vi "GaussianPeakFinder.vi"(3 "Mode":T4, 5 "Traverse line In":T1 {"Row Duration (mins)" format="%#.1f"; "Row No" min=0; "Trace Gas Concentration (%)" min=0.0 format="%#.2f"; "Emission Rate (l/min)" format="%#.2f"; "Tunnel Speed" format="%#.2f"; "Start X" format="%#.2f"; "Start Y" format="%#.2f"; "Start Z" format="%#.2f"; "End X" format="%#.2f"; "End Y" format="%#.2f"; "End Z" format="%#.2f"; "Averaging time (min)" min=0.0 format="%#.2f"}) -> (0 "Error Message":string, 1 "Status":T5, 2 "Traverse line Out":T1 {"Row Duration (mins)" format="%#.1f"; "Row No" min=0; "Trace Gas Concentration (%)" min=0.0 format="%#.2f"; "Emission Rate (l/min)" format="%#.2f"; "Tunnel Speed" format="%#.2f"; "Start X" format="%#.2f"; "Start Y" format="%#.2f"; "Start Z" format="%#.2f"; "End X" format="%#.2f"; "End Y" format="%#.2f"; "End Z" format="%#.2f"; "Averaging time (min)" min=0.0 format="%#.2f"})   [LabVIEW 2011]
uses:
  Gen Trav/Traverse_cluster.ctl
  Gen Trav/Spacing.ctl
  Controls/Multi_run_mode.ctl
  Controls/User_Specific_mode.ctl
  Gen Trav/Multi_Run_Status.ctl
  Controls/Save_Data.ctl
  Controls/Setup.ctl
  Utilities/gaussianFit/GaussianGlobal.vi
panel:
  in  "Tab Control":enum32{"GaussianFitGraph", "RunVINamed"}(tab)
  in  "nPointsInRake":i32=3
  out "nPointsSampled":i32
  in  "SpreadFactor":dbl=0.8
  in  "Turbulence":dbl=0.2
  in  "SampleLengthMultiplier":dbl=2.5
  out "MeasurementCenter":dbl
  # "X           Y            Z"
  # "Start"
  # "End"
  # "X           Y            Z"
  # "Start"
  # "End"
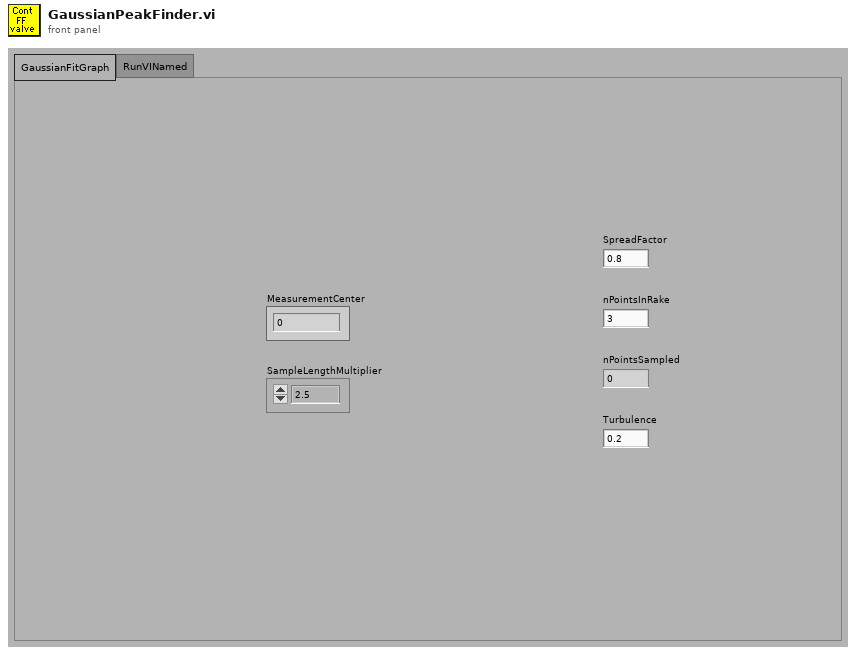
[diagram p1: front panel]
types:
  T1 = typedef "Traverse_cluster.ctl" = cluster{"Start X":dbl, "Start Y":dbl, "Start Z":dbl, "End X":dbl, "End Y":dbl, "End Z":dbl, "No. of pts.":i32, "Spacing":T2, "Filename":path, "Tunnel Speed":dbl, "Averaging time (min)":dbl, "Extra Commands":string, "Specific Arguments":string, "Emission Rate (l/min)":dbl, "Trace Gas Concentration (%)":dbl, "Density Ratio":string, "Comments":string, "Row No":i32, "Row Type Selector":T3, "Completion time":string, "Row Duration (mins)":dbl, "No. of Valid pts.":i32, "Meas Setup File":string}
  T2 = typedef "Spacing.ctl" = enum16{"Linear", "Log", "Gauss", "Specified", "N/A"}
  T3 = typedef "Multi_run_mode.ctl" = enum16{"Move Traverse Only", "Set Tunnel Speed Only", "Set Source Only", "Set Measurement Conditions", "Single Measurement", "Vertical Profile", "Lateral Profile", "Longitudinal Profile", "Explore Volume", "Multi-Axis Profile", "Auto Calibrate", "Meas Fast FID Bkgnd", "Check Beam Power", "Scanning Valve Measurement", "Run VI Named:", "Set ADAM Ch", "Wait (minutes)", "Send Message", "Synchronize With:", "Fall Back to this Row", "Turn Off Row Repeating", "Blank Row", "Traverse 3D Volume"}
  T4 = typedef "User_Specific_mode.ctl" = enum16{"Check VI only", "Run VI"}
  T5 = typedef "Multi_Run_Status.ctl" = enum16{"Continue", "Jump to Next Point", "Jump to Next Row", "Jump To Fall Back", "Terminate Run"}
  T6 = typedef "Save_Data.ctl" = enum16{"Save No Data", "Save Data"}
  T7 = typedef "Setup.ctl" = enum16{"Run Program", "Show Setup", "Save Current Setup", "Setup Front Panel"}
  T8 = typedef "Status_Cluster.ctl" = cluster{"Status":T5, "Error Type":string, "Error Description":string}
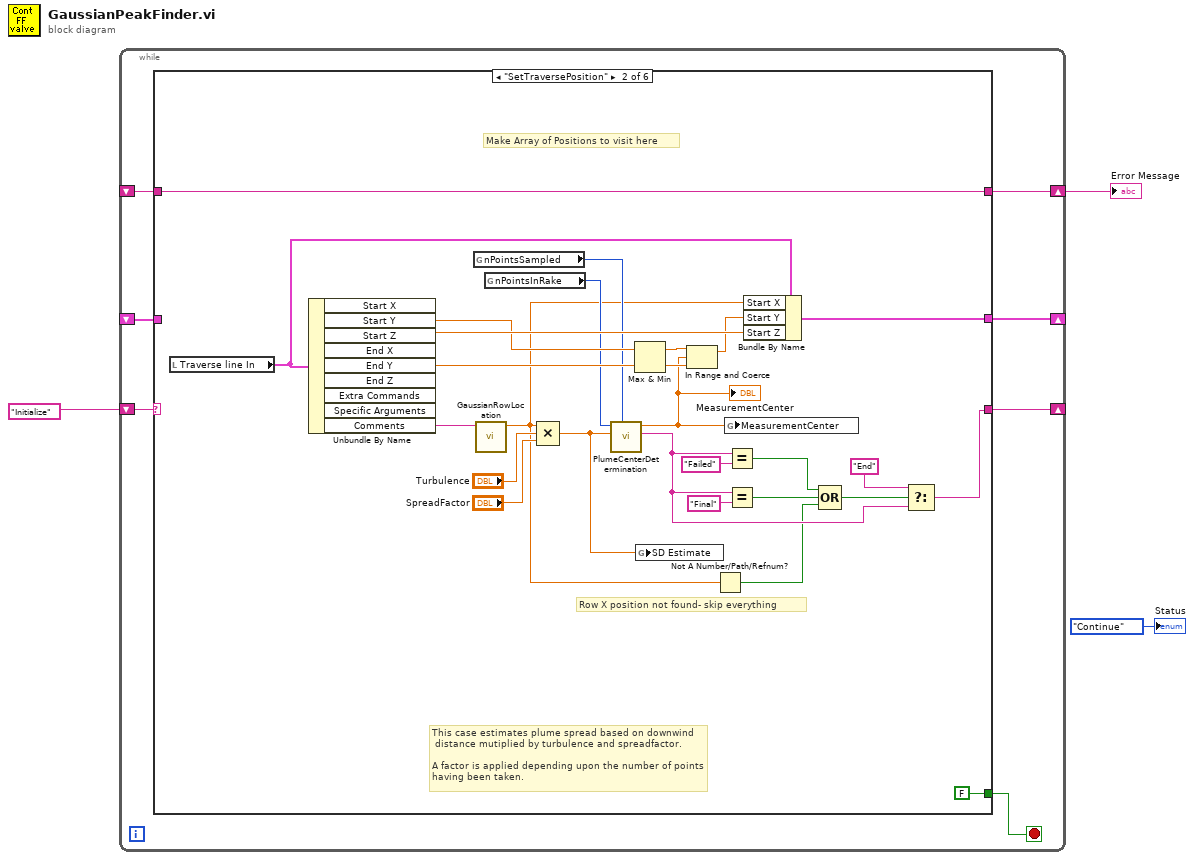
[diagram p0: block diagram]
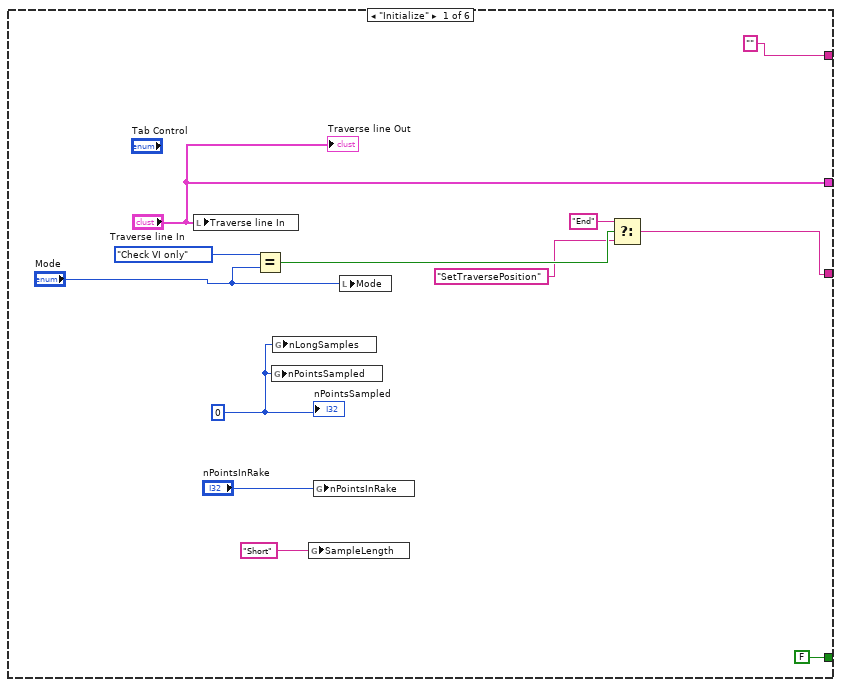
[diagram p2: hidden frame]
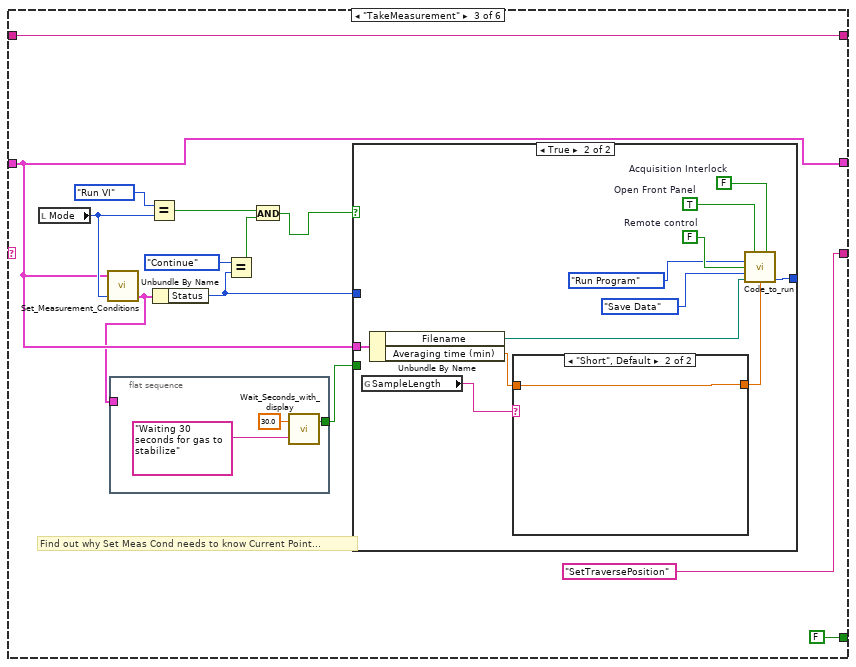
[diagram p3: hidden frame]
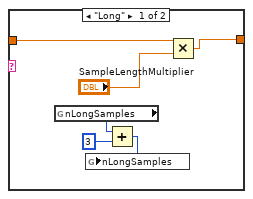
[diagram p5: hidden frame]
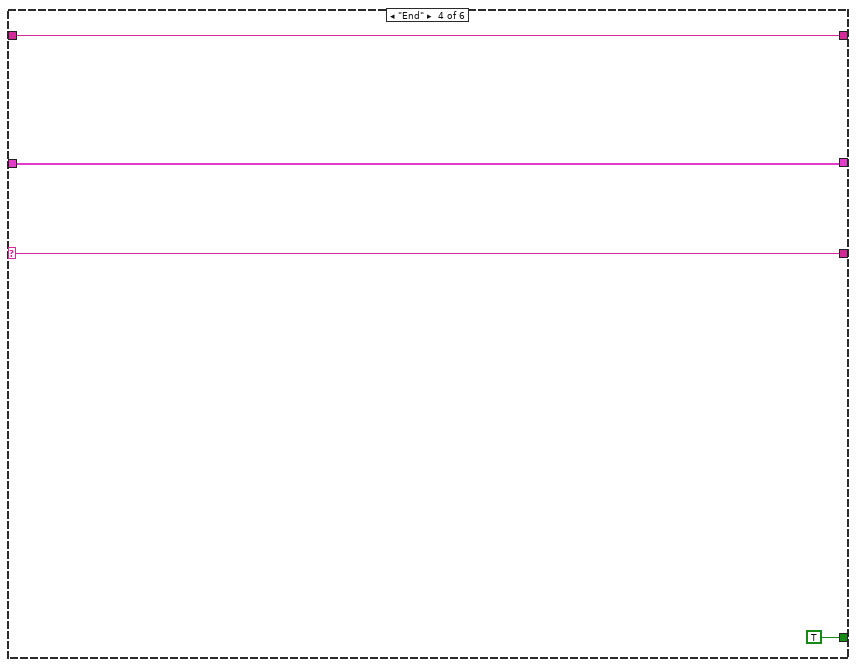
[diagram p6: hidden frame]
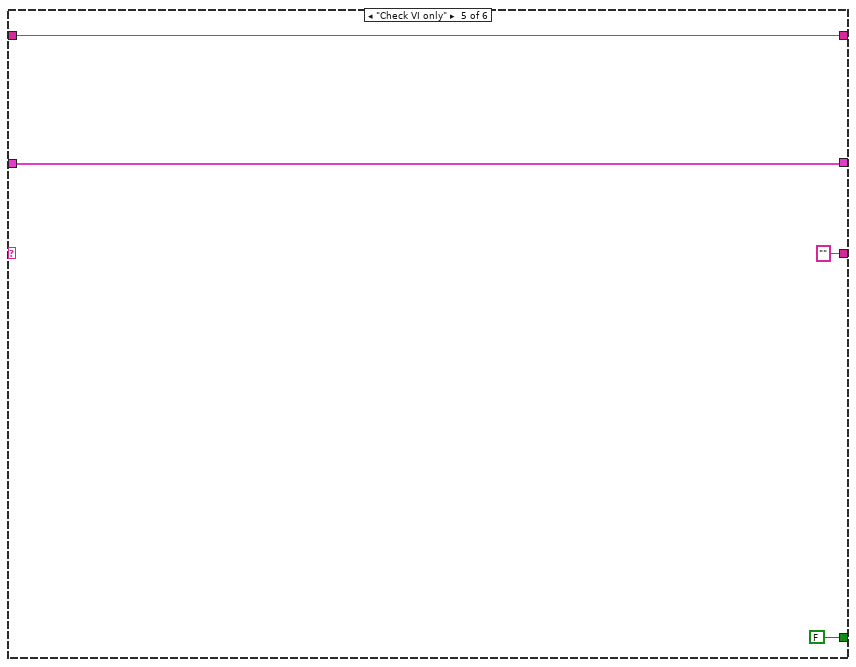
[diagram p7: hidden frame]
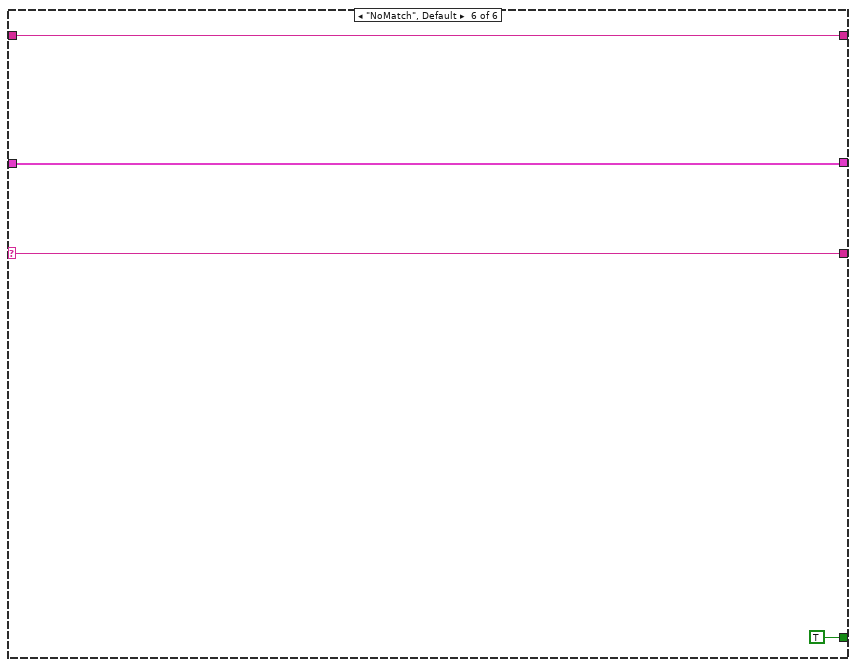
[diagram p8: hidden frame]
diagram:
  n1 = while {
    shift-right: [w8] -> _
    shift-left: _ -> [w7]
    shift-right: [w10] -> w2
    shift-left: _ -> [w5]
    shift-right: [w4] -> _
    shift-left: "Initialize" -> [w9]
    stop <- w6 stop-if-true
    n2 = case shown="\"SetTraversePosition\"" w9 {
      selector: w9 -> [_ _ _ w85 _ w93]
      tunnel: ["" w45 w56 w87 w90 w94] -> w10
      tunnel: ["Traverse line In" w48 w55 w86 w91 w95] -> w8
      tunnel: w7 -> [_ _ w55 w86 w91 w95]
      tunnel: [FALSE FALSE FALSE TRUE FALSE TRUE] -> w6
      tunnel: w5 -> [_ w45 w56 w87 w90 w94]
      tunnel: [w12 w33 "SetTraversePosition" w85 "" w93] -> w4
      frame "Initialize" {
        w18 = 0 ("PointsSampled")
        n3 = local write "Traverse line In"("Traverse line In") -> ()
        n4 = Equal?(x=User_Specific_mode."Check VI only" ("Mode 2"), y="Mode") -> (x = y?=w15:bool)
        n5 = global write "GaussianGlobal.vi" "nPointsSampled"(w18) -> ()
        n6 = global write "GaussianGlobal.vi" "nLongSamples"(w18) -> ()
        n7 = global write "GaussianGlobal.vi" "SampleLength"("Short" ("SampleLength")) -> ()
        n8 = global write "GaussianGlobal.vi" "nPointsInRake"("nPointsInRake") -> ()
        n9 = local write "Mode"("Mode") -> ()
        n10 = Select(t="End", s=w15, f="SetTraversePosition") -> (s? t:f=w12:string)
        "nPointsSampled" <- w18
        "Traverse line Out" <- "Traverse line In"
      }
      frame "SetTraversePosition" {
        # "Row X position not found- skip everything"
        # "This case estimates plume spread based on downwind\n distance mutiplied by turbulence and spreadfactor.\n\nA factor is applied depending upon the number of points\nhaving been taken."
        # "Make Array of Positions to visit here"
        n11 = local read "Traverse line In"() -> (w47:T1)
        n12 = Unbundle By Name(w47) -> ("Start Y"=w44:dbl, "Start Z"=w49:dbl, "End Y"=w43:dbl, "Comments"=w25:string)  [unwired: 5 out]
        n13 = global read "GaussianGlobal.vi" "nPointsSampled"() -> (w36:i32)
        n14 = call "GaussianRowLocation.vi"("Comments"=w25) -> ("RowXPosition"=w24:dbl)  [unwired: 10 in]
        n15 = global read "GaussianGlobal.vi" "nPointsInRake"() -> (w37:i32)
        n16 = Compound Arithmetic op=MULTIPLY(w24, "Turbulence", "SpreadFactor") -> (w31:dbl)
        n17 = call "PlumeCenterDetermination.vi"("nPointsSampled"=w36, "SD Estimate"=w31, "nPointsInRake"=w37) -> ("CommandString"=w30:string, "Measurement Center"=w32:dbl)  [unwired: 7 in]
        "MeasurementCenter" <- w32
        n18 = Max & Min(x=w44, y=w43) -> (max(x,y)=w42:dbl, min(x,y)=w41:dbl)
        n19 = global write "GaussianGlobal.vi" "SD Estimate"(w31) -> ()
        n20 = In Range and Coerce(upper limit=w42, x=w32, lower limit=w41) -> (coerced(x)=w40:dbl)  [unwired: 1 out]
        n21 = Not A Number/Path/Refnum?(number/path/refnum=w24) -> (NaN/Path/Refnum?=w23:bool)
        n22 = global write "GaussianGlobal.vi" "MeasurementCenter"(w32) -> ()
        n23 = Equal?(x=w30, y="Failed") -> (x = y?=w28:bool)
        n24 = Equal?(x=w30, y="Final") -> (x = y?=w27:bool)
        n25 = Bundle By Name(cluster=w47, "Start X"=w24, "Start Y"=w40, "Start Z"=w49) -> (w48:T1)
        n26 = Compound Arithmetic op=OR(w28, w27, w23) -> (w26:bool)
        n27 = Select(t="End" ("y"), s=w26, f=w30) -> (s? t:f=w33:string)
      }
      frame "TakeMeasurement" {
        # "Find out why Set Meas Cond needs to know Current Point..."
        n28 = local read "Mode"() -> (w58:T4)
        n29 = call "Set_Measurement_Conditions.vi"("Simulate/Run"=w58, "Traverse line"=w55) -> ("Status Cluster"=w50:T8)  [unwired: 3 in]
        n30 = flat-sequence {
          tunnel: [w65] -> w52
          tunnel: w50 -> [_]
          frame #0 {
            n31 = call "Wait_Seconds_with_display.vi"("Message"="Waiting 30 seconds for gas to stabilize", "Seconds to wait"=30.0) -> ("Stopped"=w65:bool)  [unwired: 1 in]
          }
        }
        n32 = Equal?(x=User_Specific_mode."Run VI" ("Mode"), y=w58) -> (x = y?=w62:bool)
        n33 = Unbundle By Name(w50) -> ("Status"=w53:T5)
        n34 = Equal?(x=Multi_Run_Status."Continue" ("Status"), y=w53) -> (x = y?=w59:bool)
        n35 = And(x=w62, y=w59) -> (x .and. y?=w51:bool)
        n36 = case shown="True" w51 {
          tunnel: w55 -> [_ w77]
          tunnel: w53 -> [w66 _]
          tunnel: [w66 w71] -> _
          tunnel: w52 -> [_ _]
          frame False {
          }
          frame True {
            w74 = FALSE  # Acquisition Interlock
            w75 = TRUE  # Open Front Panel
            w76 = FALSE  # Remote control
            n37 = global read "GaussianGlobal.vi" "SampleLength"() -> (w69:string)
            n38 = Unbundle By Name(w77) -> ("Filename"=w70:path, "Averaging time (min)"=w68:dbl)
            n39 = case shown="\"Short\", Default" w69 {
              tunnel: w68 -> [w83 w84]
              tunnel: [w81 w84] -> w67
              frame "Long" {
                n40 = global read "GaussianGlobal.vi" "nLongSamples"() -> (w78:i32)
                n41 = Add(x=w78, y=3) -> (x+y=w79:i32)
                n42 = global write "GaussianGlobal.vi" "nLongSamples"(w79) -> ()
                n43 = Multiply(x=w83, y="SampleLengthMultiplier") -> (x*y=w81:dbl)
              }
              frame "Short", Default {
              }
            }
            n44 = call "Code_to_run.vi"("Open Front Panel"=w75, "Acquisition Interlock"=w74, "setup"=Setup."Run Program", "Remote control"=w76, "File"=Save_Data."Save Data", "Results Filename"=w70, "Averaging time (min)"=w67) -> ("Status"=w71:T5)  [unwired: 8 in]
          }
        }
      }
      frame "End" {
      }
      frame "Check VI only" {
      }
      frame "NoMatch", Default {
      }
    }
  }
  "Error Message" <- w2
  "Status" <- Multi_Run_Status."Continue" ("Status")
